vi "PwrSwpGUI.vi"(0 "VISA IN":refnum<visa-resource-name>, 5 "error in":errorcluster={"status"=TRUE, "code"=-1073807346, "source"="VISA Clear in Initialize.vi->SystemFlush.vi->Untitled 1"}, 7 "Channel":i32=1, 9 "Port":i32=1) -> (13 "Exit":bool=TRUE, 14 "VISA Out":refnum<visa-resource-name>, 15 "Rx":string, 16 "MethodOut":string, 17 "PMET":string, 18 "MeasParameter":string, 19 "error out":errorcluster={"status"=TRUE, "code"=-1073807346, "source"="VISA Clear in Initialize.vi->SystemFlush.vi->Untitled 1"})   [LabVIEW 2018]
panel:
  in  "Meas Parameters":string="B,1"
  in  "Method":string="RPOW"
  in  "Receiver":string="POW"
  in  "Power Sensor":string="ASEN"
  in  "Power Meter Settings":string="PMET"
  in  "Offset":dbl
  in  "PwrMtr Readingds":i32=5
  in  "Settling Tolerance(dB)":dbl=0.1
  in  "Max number of readings":i32=3
  in  "Tolerance Value(dBm)":dbl=0.1
  in  "PwrMtrAdd":i32=13
  in  "Sweep Points":dbl=21.0
  in  "stop":bool
  in  "OK Button":bool
  # "Power Sweep Calibration Parameters"
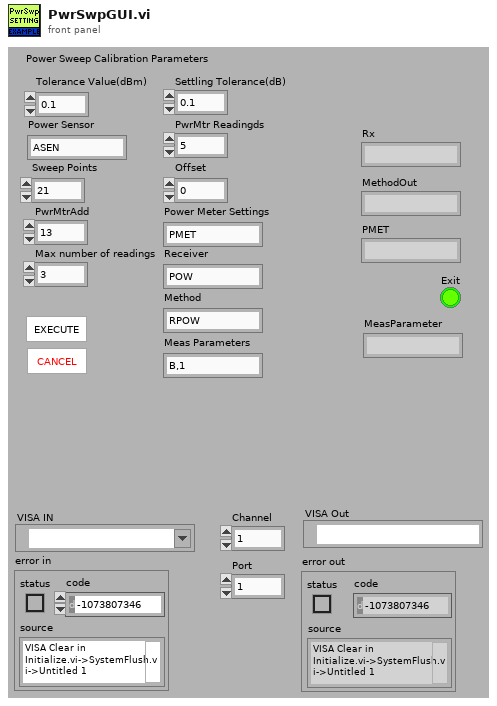
[diagram p1: front panel]
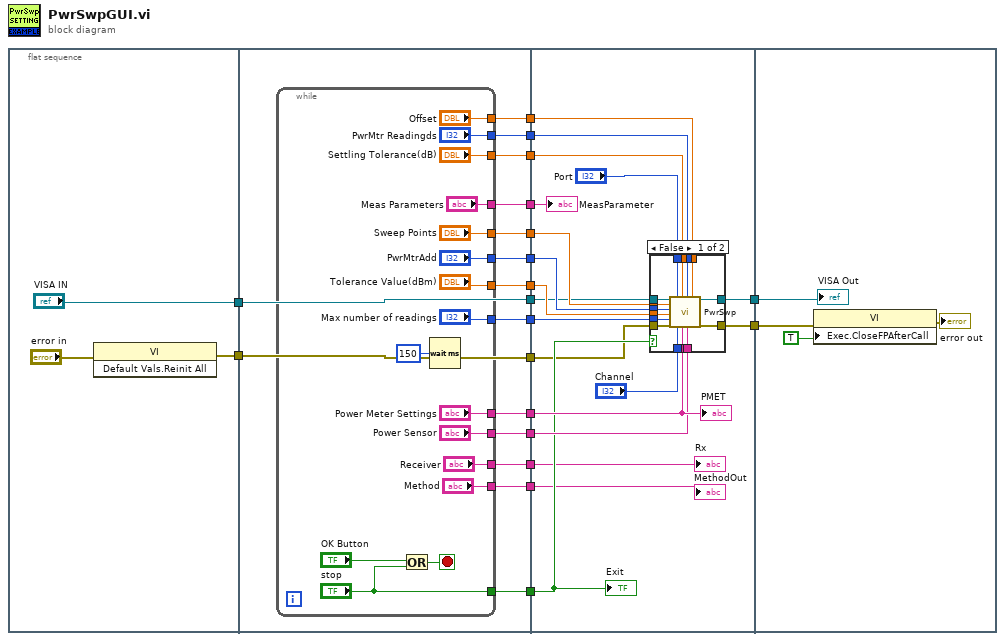
[diagram p0: block diagram]
diagram:
  n1 = flat-sequence {
    tunnel: [w21] -> w8
    tunnel: ["VISA IN"] -> w2
    tunnel: [w37] -> w19
    tunnel: [w36] -> w18
    tunnel: [w35] -> w17
    tunnel: [w34] -> w16
    tunnel: [w33] -> w15
    tunnel: [w32] -> w14
    tunnel: [w31] -> w13
    tunnel: [w30] -> w12
    tunnel: [w29] -> w11
    tunnel: [w28] -> w10
    tunnel: w8 -> [w27]
    tunnel: [w27] -> w7
    tunnel: [w26] -> w5
    tunnel: [w25] -> w4
    tunnel: [w24] -> w3
    tunnel: w2 -> [w23]
    tunnel: [w23] -> w1
    tunnel: w19 -> [w72]
    tunnel: w18 -> [w71]
    tunnel: w17 -> [w70]
    tunnel: w16 -> [w69]
    tunnel: w15 -> [w68]
    tunnel: w14 -> [w67]
    tunnel: w13 -> [w66]
    tunnel: w12 -> [w65]
    tunnel: w11 -> [w64]
    tunnel: w10 -> [w61]
    tunnel: [w60] -> w9
    tunnel: w7 -> [w59]
    tunnel: [w58] -> w6
    tunnel: w5 -> [w57]
    tunnel: w4 -> [w56]
    tunnel: w3 -> [w55]
    tunnel: w1 -> [w54]
    tunnel: w9 -> [w91]
    tunnel: w6 -> [w90]
    frame #0 {
      n2 = invoke class="VI" method="Default Vals.Reinit All"(error in="error in") -> (error out=w21:errorcluster)  [unwired: 2 in, 2 out]
    }
    frame #1 {
      n3 = while {
        tunnel: ["Offset"] -> w37
        tunnel: ["PwrMtr Readingds"] -> w36
        tunnel: ["Settling Tolerance(dB)"] -> w35
        tunnel: ["Sweep Points"] -> w34
        tunnel: ["PwrMtrAdd"] -> w33
        tunnel: ["Tolerance Value(dBm)"] -> w32
        tunnel: ["Max number of readings"] -> w31
        tunnel: ["Power Meter Settings"] -> w30
        tunnel: ["Power Sensor"] -> w29
        tunnel: ["stop"] -> w28
        tunnel: ["Receiver"] -> w26
        tunnel: ["Method"] -> w25
        tunnel: ["Meas Parameters"] -> w24
        stop <- w53 stop-if-true
        n4 = Or(x="OK Button", y="stop") -> (x .or. y?=w53:bool)
        n5 = Wait (ms)(milliseconds to wait=u32 150) -> ()  [unwired: 1 out]
      }
    }
    frame #2 {
      n6 = case shown="False" w61 {
        tunnel: w72 -> [w87 _]
        tunnel: w71 -> [w86 _]
        tunnel: w70 -> [w85 _]
        tunnel: w69 -> [w84 _]
        tunnel: w68 -> [w83 _]
        tunnel: w67 -> [w82 _]
        tunnel: w66 -> [w81 _]
        tunnel: w65 -> [w80 _]
        tunnel: w64 -> [w79 _]
        tunnel: w59 -> [w78 w89]
        tunnel: "Channel" -> [w77 _]
        tunnel: "Port" -> [w76 _]
        tunnel: [w75 w88] -> w58
        tunnel: [w74 w89] -> w60
        tunnel: w54 -> [w73 w88]
        frame False {
          n7 = call "PwrSwp.vi"("VISA IN"=w73, "Sweep Points"=w84, "PwrMtrAdd"=w83, "Tolerance Value(dBm)"=w82, "Max number of readings"=w81, "error in"=w78, "Port"=w76, "Channel"=w77, "Settling Tolerance(dB)"=w85, "Power Meter Settings"=w80, "PwrMtr Readingds"=w86, "Power Sensor"=w79, "Offset"=w87) -> ("VISA Out"=w75:refnum<visa-resource-name>, "error out"=w74:errorcluster)  [unwired: 5 in]
        }
        frame True {
        }
      }
      "Exit" <- w61
      "PMET" <- w65
      "Rx" <- w57
      "MethodOut" <- w56
      "MeasParameter" <- w55
    }
    frame #3 {
      n8 = property class="VI"(error in=w91, "Exec.CloseFPAfterCall"=TRUE ("Execution:Close After Call")) -> (error out=→"error out":errorcluster)  [unwired: 1 in, 1 out]
      "VISA Out" <- w90
    }
  }
